vi "amy_test.vi"() -> ()   [LabVIEW 2017]
panel:
  out "Waveform Chart":dbl(graph)
  in  "Slide 2":dbl(slide) scale=0.0..10.0
  in  "Slide":dbl(slide) scale=0.0..10.0
  in  "Filename":path=path "test.tdms"
  out "Thermocouples \n(Celsius)":dbl[](array[numeric])
  in  "stop 2":bool
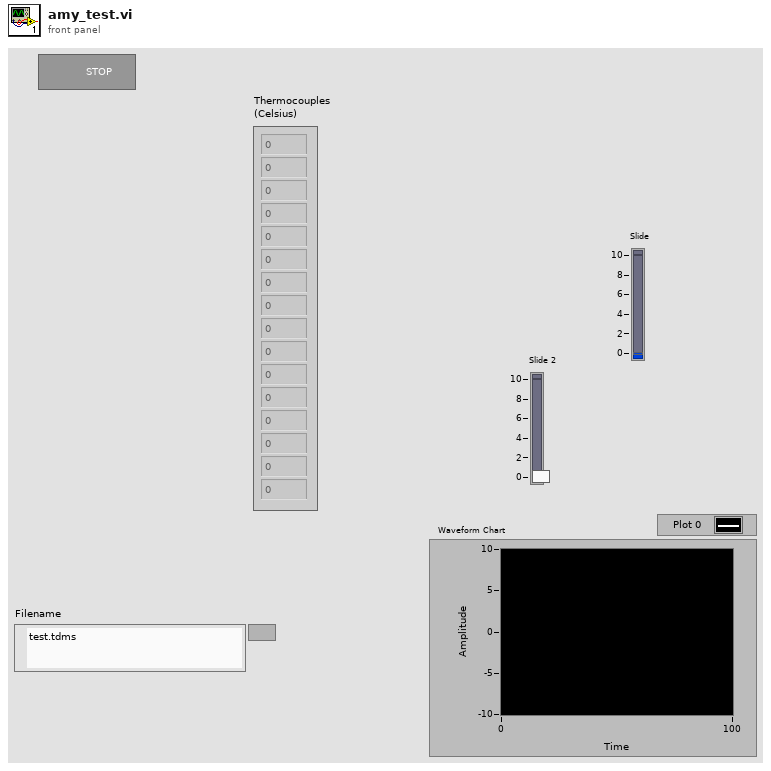
[diagram p1: front panel]
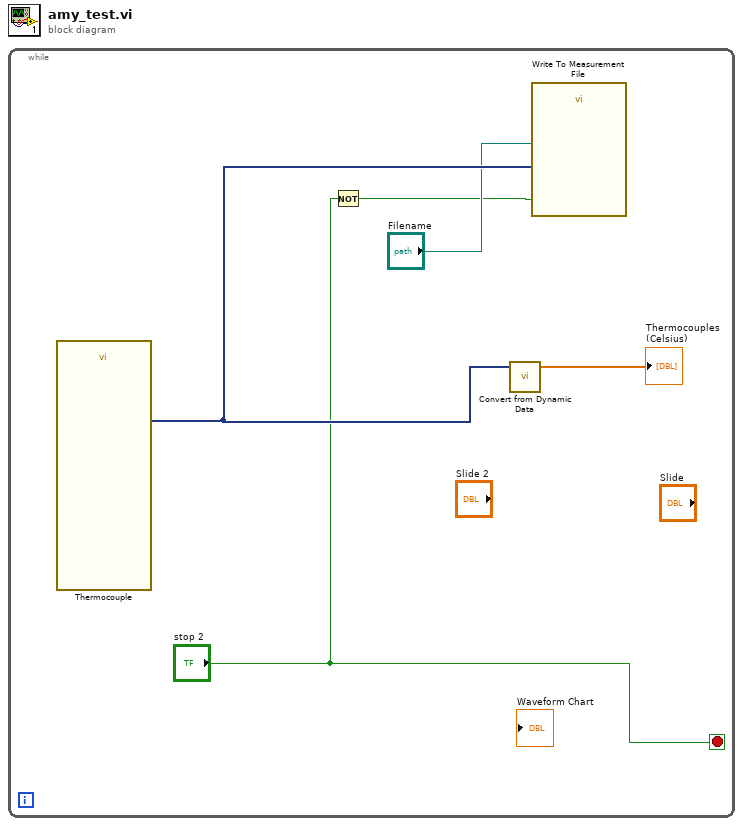
[diagram p0: block diagram]
diagram:
  n1 = while {
    stop <- "stop 2" stop-if-true
    n2 = call "Thermocouple"() -> ("data"=w4:dynamicdata)  [unwired: 16 in, 3 out]
    n3 = Not(x="stop 2") -> (.not. x?=w1:bool)
    n4 = call "Convert from Dynamic Data"("Dynamic Data Type"=w4) -> ("Array"=→"Thermocouples \n(Celsius)":dbl[])  [unwired: 3 in]
    n5 = call "Write To Measurement File"("Signals"=w4, "Flush? (T)"=w1, "Filename"="Filename") -> ()  [unwired: 14 in, 3 out]
  }
